vi "launcher.vi"   [LabVIEW 2023]
uses:
  Camera_Controller/Camera_Controller.lvclass
  <vilib>/ActorFramework/Actor/Actor.lvclass
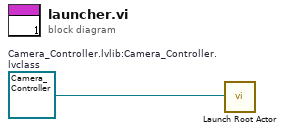
[diagram p0: block diagram]
diagram:
  w1 = refnum<class "Camera_Controller.lvclass"> refnum  # Camera_Controller.lvlib:Camera_Controller.lvclass
  n1 = call <vilib>:"Launch Root Actor.vi"("Actor"=w1) -> ()  [unwired: 9 in, 2 out]
